vi "Main.vi"(11 "Module Admin":refnum<class "Delacor_lib_QMH_Module Admin.lvclass">) -> ()   [LabVIEW 2023, in "Panther Dashboard.lvlib"]
doc: "Panther Dashboard For DQMH®\n\nDeveloped and maintained by:\nPantherLAB\n\nMain Contributor- Developer:\n\n» Enrique Noé Arias\n\nBrainstorming & Code Reviews:\n\n» Matthias Baudot\n» Fabiola De La Cueva\n» Christopher Farmer\n» Cyril Gambini\n» Joerg Hampel\n» Olivier Jourdan\n» Cesar Muñoz\n» Darren Nattinger\n» Luis Orozco\n» Sam Taggart\n» Diego Torres"
uses:
  Panther Dashboard.lvlib
  <vilib>/Delacor/Delacor QMH/Libraries/Module Admin_class/Delacor_lib_QMH_Module Admin.lvclass
  Module Data--cluster.ctl
  Maps List and refs--cluster.ctl
  <vilib>/National Instruments/Tree Map/Tree Map Data.ctl
  DQMH Modules Info--cluster.ctl
  Module type--enum.ctl
  Project References--cluster.ctl
  Selection Type--enum.ctl
  References Updated Argument--cluster.ctl
  Launch DQMH Scripting Tools Argument--cluster.ctl
  DQMH Tools Menu--enum.ctl
  <vilib>/Delacor/Delacor QMH/Libraries/Message Queue_class/Delacor_lib_QMH_Message Queue.lvclass/Delacor_lib_QMH_Message Queue.ctl
  Expand Results Argument--cluster.ctl
  Execute Default Event Request Argument--cluster.ctl
  Tree DQMH Selection Argument--cluster.ctl
  Scan DQMH Modules Argument--cluster.ctl
  Stop Argument--cluster.ctl
  Generate Project Documentation Argument--cluster.ctl
  Set App Theme Argument--cluster.ctl
  Show About Argument--cluster.ctl
  Update Module ID Argument--cluster.ctl
  Save Library Description Argument--cluster.ctl
  Save VI Description Argument--cluster.ctl
  Open Documentation Argument--cluster.ctl
  Save Project Documentation Argument--cluster.ctl
  Public VIs names--enum.ctl
  <vilib>/Delacor/Delacor QMH/Libraries/Module Admin_class/Delacor_lib_QMH_Module Admin.lvclass/Delacor_lib_QMH_Module Admin.ctl
  <vilib>/Delacor/Delacor QMH/Libraries/Message Queue_class/Delacor_lib_QMH_Enqueue Message (Single).vi
  <vilib>/Delacor/Delacor QMH/Libraries/Module Admin_class/Delacor_lib_QMH_Get External Launch.vi
  Panther Dashboard--global.vi
  <vilib>/National Instruments/Tree Map/API/List Roots.vi
  <vilib>/National Instruments/Tree Map/Utility/Into Tree Control Items.vi
  <vilib>/Utility/error.llb/Error Cluster From Error Code.vi
  <vilib>/ErrorRing/Error Ring.xnode
  <vilib>/Delacor/Delacor QMH/Libraries/Message Queue_class/Delacor_lib_QMH_Message Queue.lvclass
  <vilib>/National Instruments/Tree Map/Tree Map.lvlib
  <vilib>/Delacor/Delacor QMH/Libraries/Scripting API/DQMH_Scripting API.lvlib
  ContextHelp/ContextHelp.lvlib
panel:
  out "error out":errorcluster
  in  "Context Help Panther":bool caption="Doc Editor"
  in  "Add Event":bool
  in  "Remove Event":bool caption="Remove"
  in  "Convert Event":bool caption="Convert"
  in  "Rename Event":bool caption="Rename"
  in  "Add New Module":bool caption="Add"
  in  "Rename Module":bool caption="Rename"
  in  "Validate Module":bool caption="Validate"
  in  "Create Module Template":bool caption="Template"
  in  "Add Unit Test Module":bool caption="Unit Test"
  in  "Create RT Tester Module":bool caption="RT Tester"
  in  "About Panther":bool caption="About"
  in  "Theme Panther":bool caption="Theme"
  in  "Projects":string(combo)
  in  "Targets":string(combo)
  in  "Search":bool caption="Scan Project"
  in  "Expand Results":bool
  in  "Include Dependencies":bool
  in  "Module ID":i32=-1 min=-1 max=1000 step=1 format="Module ID %d"
  in  "Modules Tree":string(tree) caption="Tree 2"
  out "Panther Indicator":bool
  out "Process Indicator":bool
  out "Event Indicator":bool
  out "Status":string
  out "Progress":u16(slide) scale=-1.0..4.0
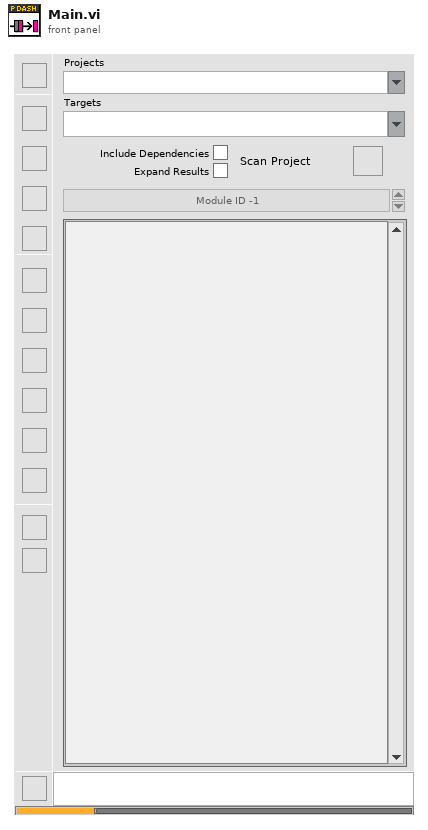
[diagram p1: front panel]
types:
  T1 = typedef "Panther Dashboard.lvlib/Broadcast Events--cluster.ctl" = cluster{"Module Did Init":refnum<user-event>, "Status Updated":refnum<user-event>, "Error Reported":refnum<user-event>, "Module Did Stop":refnum<user-event>, "Update Module Execution Status":refnum<user-event>, "References Updated":refnum<user-event>, "Projects Updated":refnum<user-event>, "Targets Updated":refnum<user-event>, "Progress updated":refnum<user-event>, "Scale Updated":refnum<user-event>, "Connector Pane Updated":refnum<user-event>, "Documentation Updated":refnum<user-event>, "Module Type Updated":refnum<user-event>, "Theme Updated":refnum<user-event>, "Project Description Updated":refnum<user-event>}
  T2 = typedef "Panther Dashboard.lvlib/Request Events--cluster.ctl" = cluster{"Stop Module":refnum<user-event>, "Show Panel":refnum<user-event>, "Hide Panel":refnum<user-event>, "Get Module Execution Status":refnum<user-event>, "Show Diagram":refnum<user-event>, "Scan DQMH Modules":refnum<user-event>, "Tree DQMH Selection":refnum<user-event>, "Open Module API Tester":refnum<user-event>, "Execute Default Event Request":refnum<user-event>, "Expand Results":refnum<user-event>, "Launch DQMH Scripting Tools":refnum<user-event>, "Generate Project Documentation":refnum<user-event>, "Set App Theme":refnum<user-event>, "Show About":refnum<user-event>, "Update Module ID":refnum<user-event>, "Save Library Description":refnum<user-event>, "Save VI Description":refnum<user-event>, "Open Documentation":refnum<user-event>, "Save Project Documentation":refnum<user-event>, "Register controls Mouse Enter":refnum<user-event>}
  T3 = typedef "ContextHelp.lvlib/Broadcast Events--cluster.ctl" = cluster{"Module Did Init":refnum<user-event>, "Status Updated":refnum<user-event>, "Error Reported":refnum<user-event>, "Module Did Stop":refnum<user-event>, "Update Module Execution Status":refnum<user-event>}
  T4 = typedef "Panther Dashboard.lvlib/Selection Type--enum.ctl" = enum16{"Broadcast", "Request", "Module", "Public API"}
  T5 = typedef "Panther Dashboard.lvlib/Module Data--cluster.ctl" = cluster{"Maps":T6, "DQMH Scan Results":T8, "Current Selection":cluster{"VI Ref":refnum<vi>, "DQMH Lib Ref":refnum<vi>}, "Module type":T9, "Module ID":i32, "Theme":bool, "Broadcast?":bool}
  T6 = typedef "Panther Dashboard.lvlib/Maps List and refs--cluster.ctl" = cluster{"Tree Map":T7, "References Map":map{string, refnum<vi>}}
  T7 = typedef "Tree Map.lvlib/Tree Map Data.ctl" = map{string, cluster{"Child Paths Set":set{string}, "Name":string, "Data":string, "Attributes":map{string, string}}}
  T8 = typedef "Panther Dashboard.lvlib/DQMH Modules Info--cluster.ctl" = cluster{"All DQMH Modules Refs":refnum<vi>[], "All Modules Descriptions":string[], "All Modules type":T9[], "Project References":T10}
  T9 = typedef "Panther Dashboard.lvlib/Module type--enum.ctl" = enum16{"Module type: Singleton", "Module type: Cloneable"}
  T10 = typedef "Panther Dashboard.lvlib/Project References--cluster.ctl" = cluster{"Project Ref":refnum<vi>, "Project Name":string, "Target":refnum<vi>, "App Ref":refnum<vi>}
  T11 = typedef "Panther Dashboard.lvlib/References Updated Argument--cluster.ctl" = cluster{"Modules":refnum<vi>[], "Modules Types":T9[], "Application Instance":refnum<vi>}
  T12 = enum8{"Enabled", "Disabled", "Disabled and Grayed Out"}
  T13 = typedef "Panther Dashboard.lvlib/Launch DQMH Scripting Tools Argument--cluster.ctl" = cluster{"Scripting Tool":T14}
  T14 = typedef "Panther Dashboard.lvlib/DQMH Tools Menu--enum.ctl" = enum16{"Create New DQMH Event", "Remove DQMH Event", "Convert DQMH Event", "Rename DQMH Event", "Add New DQMH Module", "Create RT Tester", "Rename DQMH Module", "Validate DQMH Module", "Create DQMH Module Template", "New DQMH  Unit Test"}
  T15 = typedef "Panther Dashboard.lvlib/Expand Results Argument--cluster.ctl" = cluster{"Expand?":bool}
  T16 = typedef "Panther Dashboard.lvlib/Execute Default Event Request Argument--cluster.ctl" = cluster{"Event Name":string}
  T17 = typedef "Panther Dashboard.lvlib/Tree DQMH Selection Argument--cluster.ctl" = cluster{"Tree DQMH Sel":string}
  T18 = typedef "Panther Dashboard.lvlib/Scan DQMH Modules Argument--cluster.ctl" = cluster{"Include Dependencies":bool, "Project":string, "Target":string}
  T19 = enum32{"invalid lock state", "Not Locked", "Locked (No Password)", "Password-protected"}
  T20 = typedef "Panther Dashboard.lvlib/Stop Argument--cluster.ctl" = cluster{"Origin":string, "Exit via Stop Module Req?":bool, "Wait for Module to stop?":bool}
  T21 = typedef "Panther Dashboard.lvlib/Generate Project Documentation Argument--cluster.ctl" = cluster{"Boolean":bool}
  T22 = typedef "Panther Dashboard.lvlib/Set App Theme Argument--cluster.ctl" = cluster{"Theme":bool}
  T23 = typedef "Panther Dashboard.lvlib/Show About Argument--cluster.ctl" = cluster{"Boolean":bool}
  T24 = typedef "Panther Dashboard.lvlib/Update Module ID Argument--cluster.ctl" = cluster{"New ID":i32}
  T25 = typedef "Panther Dashboard.lvlib/Save Library Description Argument--cluster.ctl" = cluster{"Library Description":string}
  T26 = typedef "Panther Dashboard.lvlib/Save VI Description Argument--cluster.ctl" = cluster{"VI Description":string}
  T27 = typedef "Panther Dashboard.lvlib/Open Documentation Argument--cluster.ctl" = cluster{"Boolean":bool}
  T28 = typedef "Panther Dashboard.lvlib/Save Project Documentation Argument--cluster.ctl" = cluster{"Project Description":string}
  T29 = typedef "Panther Dashboard.lvlib/Public VIs names--enum.ctl" = enum16{"Start Module.vi", "Synchronize Module Events.vi", "Obtain Broadcast Events for Registration.vi", "Null Broadcast Events--constant.vi", "Stop Module.vi"}
  T30 = cluster{"Left Cell String":string, "Child Text":string[], "Child Tag":string, "Item Indent":i32, "Child Only?":bool, "Glyph Index":i32}[]
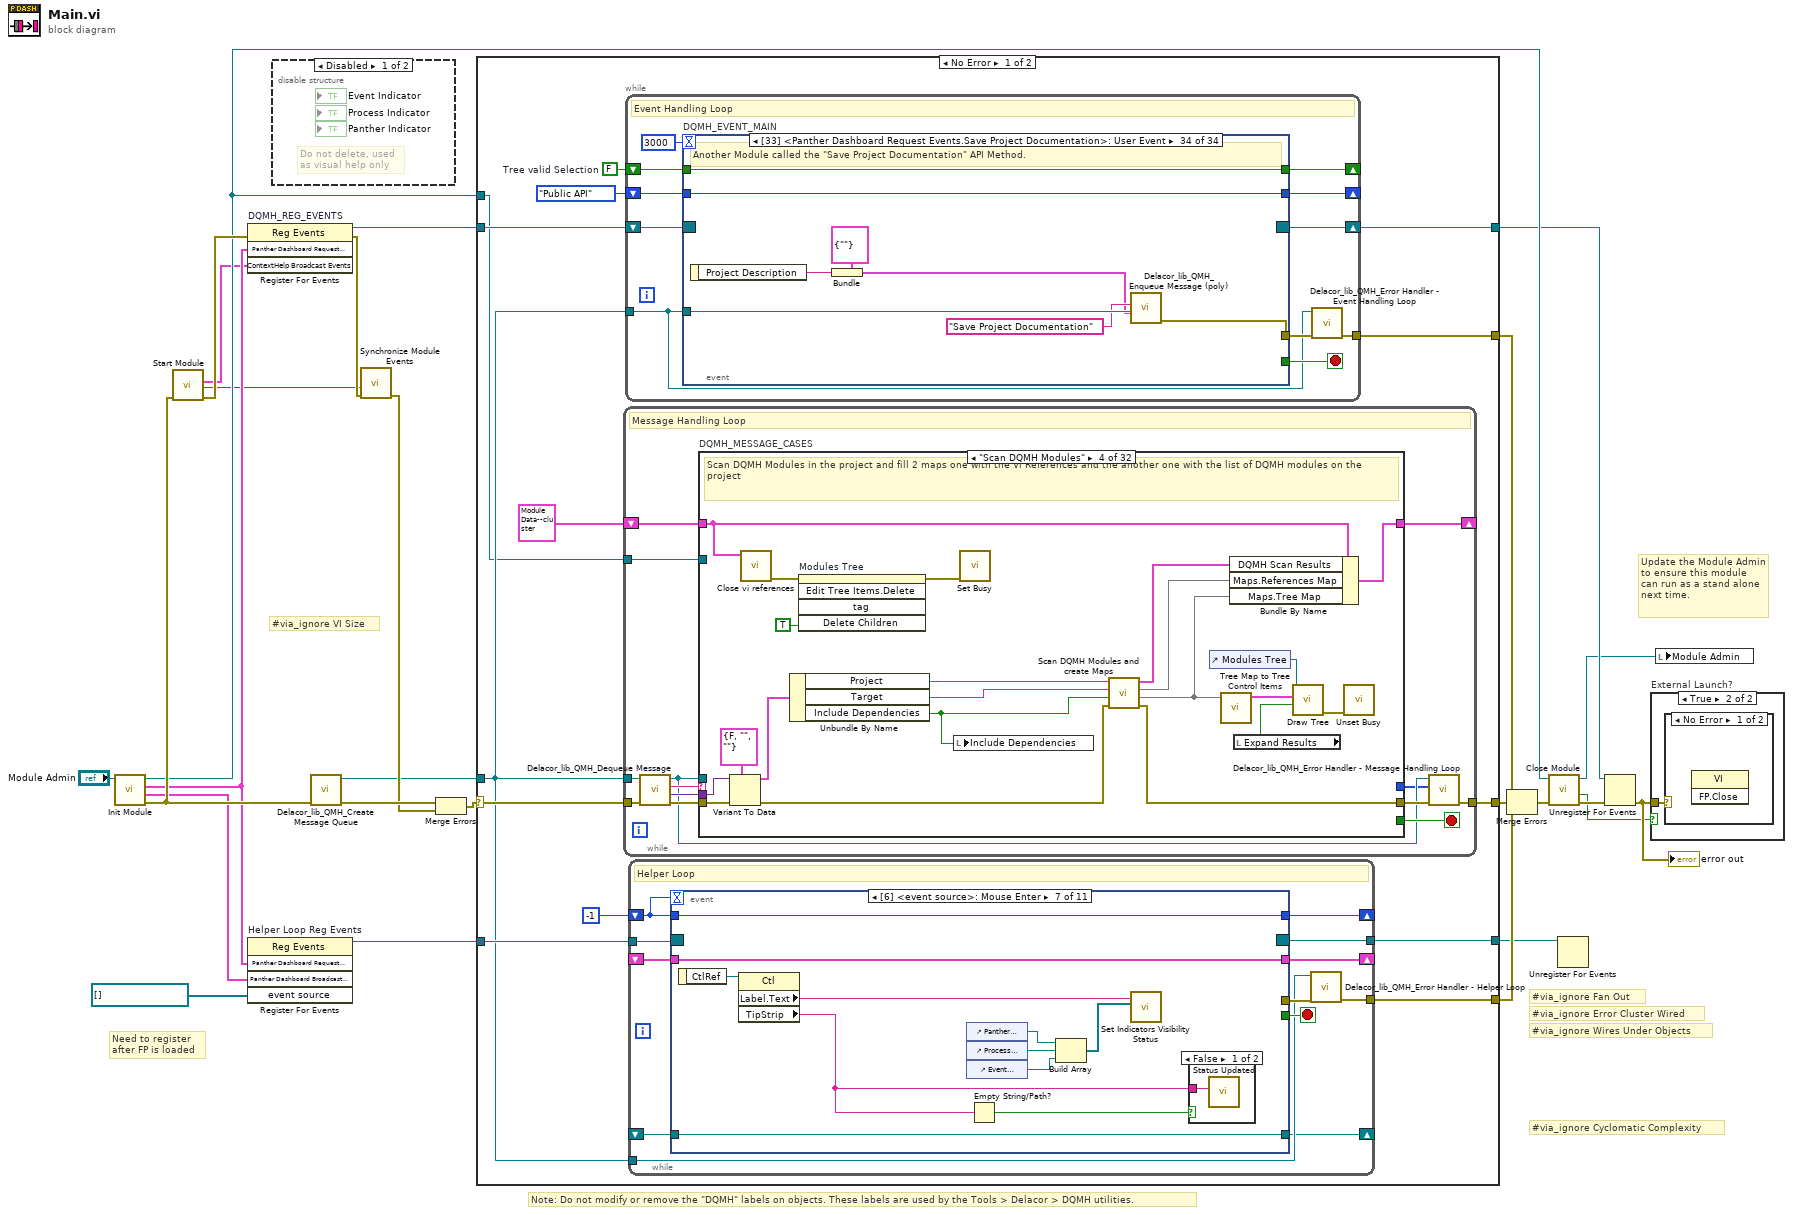
[diagram p0: block diagram]
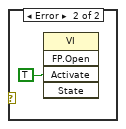
[diagram p4: hidden frame]
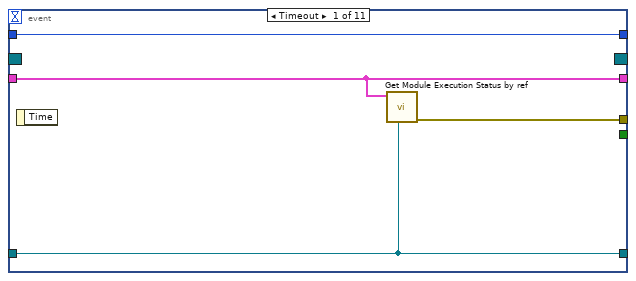
[diagram p5: hidden frame]
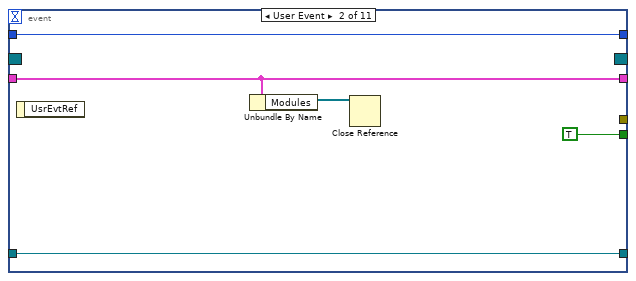
[diagram p6: hidden frame]
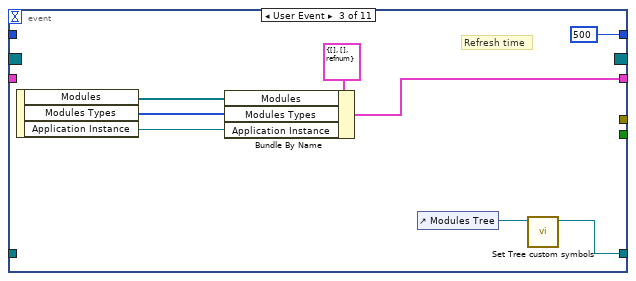
[diagram p7: hidden frame]
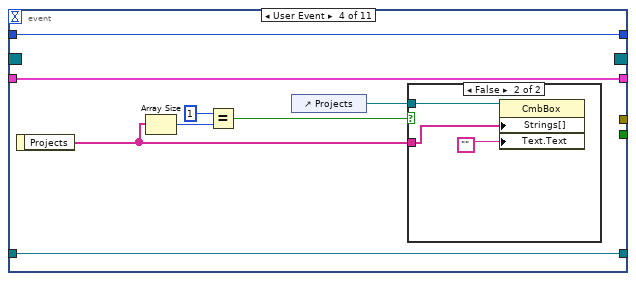
[diagram p8: hidden frame]
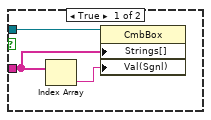
[diagram p9: hidden frame]
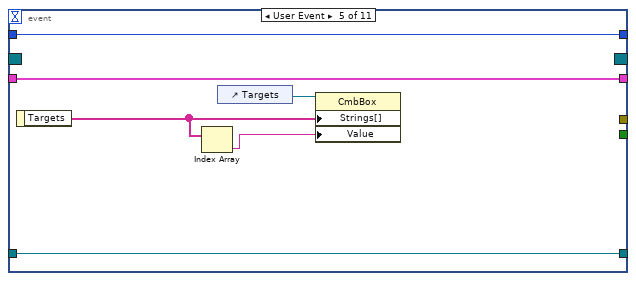
[diagram p10: hidden frame]
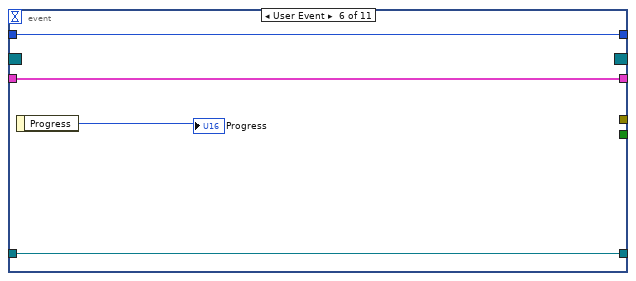
[diagram p11: hidden frame]
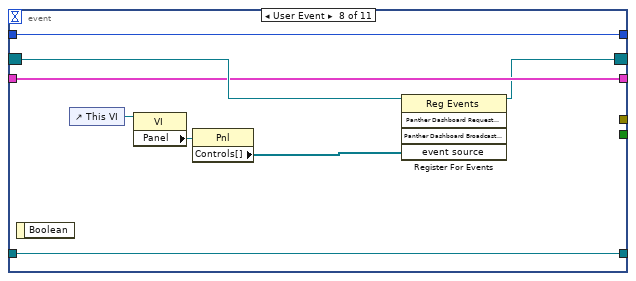
[diagram p13: hidden frame]
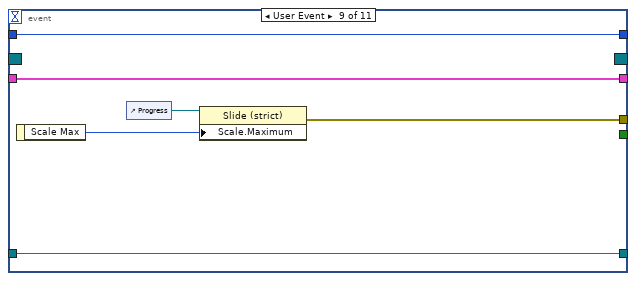
[diagram p14: hidden frame]
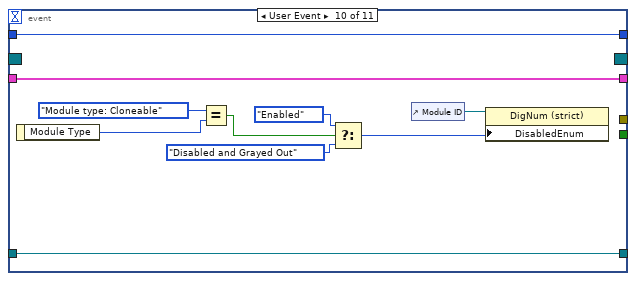
[diagram p15: hidden frame]
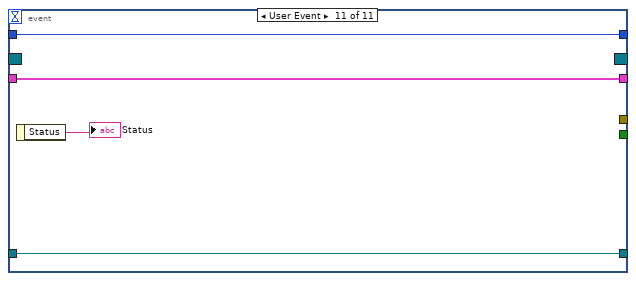
[diagram p16: hidden frame]
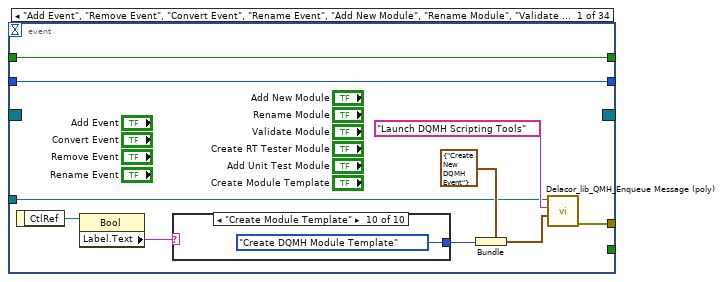
[diagram p17: hidden frame]
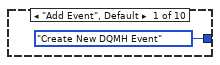
[diagram p18: hidden frame]
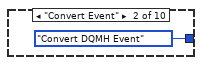
[diagram p19: hidden frame]
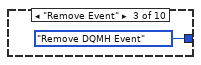
[diagram p20: hidden frame]
diagram:
  # "Need to register\nafter FP is loaded"
  # "#via_ignore VI Size"
  # "#via_ignore Fan Out"
  # "#via_ignore Cyclomatic Complexity"
  # "#via_ignore Wires Under Objects"
  # "#via_ignore Error Cluster Wired"
  # "Note: Do not modify or remove the \"DQMH\" labels on objects. These labels are used by the Tools > Delacor > DQMH utilities."
  # "Update the Module Admin to ensure this module can run as a stand alone next time."
  n1 = call "Init Module.vi"("Singleton Module Admin in"="Module Admin") -> ("error out"=w15:errorcluster, "Panther Dashboard Broadcast Events"=w4:T1, "Panther Dashboard Request Events"=w5:T2, "Singleton Module Admin out"=w14:refnum<class "Delacor_lib_QMH_Module Admin.lvclass">)  [unwired: 7 in]
  n2 = call "Start Module.vi"("error in"=w15) -> ("error out"=w17:errorcluster, "Wait for Event Sync?"=w3:bool, "ContextHelp Broadcast Events"=w2:T3)  [unwired: 7 in, 1 out]
  n3 = register-events "DQMH_REG_EVENTS"(error in=w17, w5, w2) -> (reference out=w12:refnum<event-registration>, error out=w18:errorcluster)  [unwired: 1 in]
  n4 = register-events "Helper Loop Reg Events"(w5, w4, refnum<vi>[] [] ("event source")) -> (reference out=w7:refnum<event-registration>)  [unwired: 2 in, 1 out]
  n5 = disable-structure shown="Disabled" {
    frame Disabled {
      # "Do not delete, used\nas visual help only"
    }
    frame Enabled {
    }
  }
  n6 = call <vilib>:"Delacor_lib_QMH_Create Message Queue.vi"("error in"=w15) -> ("error out"=w21:errorcluster, "Message Queue"=w11:refnum<class "Delacor_lib_QMH_Message Queue.lvclass">)  [unwired: 9 in]
  n7 = call "Synchronize Module Events.vi"("error in"=w18, "Wait for Event Sync?"=w3) -> ("error out"=w16:errorcluster)  [unwired: 9 in]
  n8 = Merge Errors(w21, w16) -> (w20:errorcluster)
  n9 = case shown="No Error" w20 {
    selector: w20 -> [w38 w777]
    tunnel: [w40 w776] -> w26
    tunnel: [w36 w775] -> w13
    tunnel: w12 -> [w34 w775]
    tunnel: w11 -> [w30 w771]
    tunnel: [w39 _] -> w24
    tunnel: w14 -> [w27 w772]
    tunnel: w7 -> [w33 w770]
    tunnel: [w32 w770] -> w6
    tunnel: [w37 _] -> w19
    frame No Error {
      w29 = FALSE  # Tree valid Selection
      n10 = while {
        tunnel: w30 -> [w428]
        shift-right: [w432] -> _
        shift-left: T5 {"Maps"={"Tree Map"={}, "References Map"={}}, "DQMH Scan Results"={"All DQMH Modules Refs"=[], "All Modules Descriptions"=[], "All Modules type"=[], "Project References"={"Project Ref"=refnum, "Project Name"="", "Target"=refnum, "App Ref"=refnum}}, "Current Selection"={"VI Ref"=refnum, "DQMH Lib Ref"=refnum}, "Module type"=enum."Module type: Singleton", "Module ID"=0, "Theme"=FALSE, "Broadcast?"=FALSE} ("Data Cluster") -> [w433]
        tunnel: w38 -> [w436]
        tunnel: [w434] -> w40
        tunnel: w27 -> [w426]
        stop <- w431 stop-if-true
        # "Message Handling Loop"
        n11 = call-dynamic "Delacor_lib_QMH_Dequeue Message.vi"("error in"=w436, "Message Queue in"=w428) -> ("error out"=w435:errorcluster, "Message Data"=w429:variant, "Message"=w430:string, "Message Queue out"=w427:refnum<class "Delacor_lib_QMH_Message Queue.lvclass">)  [unwired: 6 in]
        n12 = case "DQMH_MESSAGE_CASES" shown="\"Scan DQMH Modules\"" w430 {
          selector: w430 -> [_ w465 _ _ _ _ _ _ _ _ _ _ _ _ _ _ _ _ _ _ _ _ _ _ _ _ _ _ _ _ _ w756]
          tunnel: w427 -> [_ _ _ _ _ _ _ _ _ _ _ _ _ _ _ _ _ _ _ _ _ _ _ _ _ _ _ _ _ w725 w748 _]
          tunnel: w435 -> [w459 w470 w472 w493 w500 w507 w514 w521 w536 w545 w550 w556 w570 w583 w605 w611 w613 w625 w632 w637 w650 w661 w670 w678 w688 w704 w717 w720 w722 w732 w754 w758]
          tunnel: [w453 w468 w472 w492 w499 w507 w514 w521 w535 w544 w551 w557 w568 w581 w606 w610 w614 w624 w631 w636 w648 w658 w666 w677 w686 w702 w715 w719 w722 w728 w751 w759] -> w437
          tunnel: w433 -> [w438 w467 w471 w479 w497 w506 w513 w520 w531 w543 w549 w555 w563 w580 w604 w609 w618 w623 w630 w635 w639 w657 w665 w676 w680 w697 w711 w718 w721 w727 w740 w757]
          tunnel: [w450 w467 w471 w484 w497 w506 w513 w520 w527 w543 w549 w555 w563 w580 w604 w609 w618 w621 w630 w635 w639 w652 w665 w672 w679 w695 w711 w718 w721 w727 w740 w757] -> w432
          tunnel: [_ _ _ _ _ _ _ _ _ _ _ _ _ _ _ _ _ _ _ _ _ _ _ _ _ _ _ _ _ _ w747 _] -> w431
          tunnel: w429 -> [_ w466 _ w487 _ _ _ _ w534 _ _ _ w566 _ _ _ _ w622 w629 _ w647 w656 w664 w675 w684 w700 w714 _ _ w726 w746 _]
          tunnel: w426 -> [w451 _ _ _ _ _ _ _ _ _ _ _ _ _ _ _ _ _ _ _ _ _ _ _ _ _ _ _ _ w724 w741 _]
          tunnel: [_ _ _ _ _ _ _ _ _ _ _ _ _ i32[] [5000, 1026, 43] ("specific error code to clear (0: all)") _ _ _ _ _ _ _ _ _ _ _ _ _ _ _ _ _ _] -> w425
          frame "Initialize" {
            w441 = "Panther Dashboard for DQMH" ("format string")
            # "Initialize - Any operation that needs to be done before the module can receive messages. Synchronize Caller Events.vi will inform Start Module.vi that the module has launched and is ready to receive messages. Module Did Init.vi will broadcast that the module initialized."
            n13 = call "Synchronize Caller Events.vi"("error in (no error)"=w459, "Singleton Module Admin in"=w451) -> ("error out"=w458:errorcluster)  [unwired: 8 in, 1 out]
            n14 = call "Module Name--constant.vi"() -> ("Module Name"=w448:string)  [unwired: 11 in]
            n15 = disable-structure shown="Disabled" {
              disable-tunnel: [w462 _] -> w439
              disable-tunnel: w438 -> [w461 _]
              frame Disabled {
                n16 = call "Close vi references.vi"("Data Cluster"=w461) -> ("error out"=w460:errorcluster)  [unwired: 10 in]
                n17 = invoke on="Modules Tree" class="Tree (strict)" method="Edit Tree Items.Delete"(error in=w460) -> (error out=w462:errorcluster)  [unwired: 4 in, 4 out]
              }
              frame Enabled {
              }
            }
            n18 = call "Module Did Init.vi"("error in (no error)"=w458, "Initialized?"=TRUE, "Origin"=w448) -> ("error out"=w457:errorcluster)  [unwired: 8 in]
            n19 = property on="Modules Tree" class="Tree (strict)"(error in=w439, "Allow Item Drag"=TRUE ("Drag/Drop:Allow Dragging"), "SelColor"=u32 8355711) -> ()  [unwired: 1 in, 2 out]
            n20 = control-ref of="Projects"() -> (w444:refnum<vi>)
            n21 = call "Scan For App Projects.vi"("error in"=w457, "Init?"=TRUE, "Projects Ref"=w444) -> ("error out"=w456:errorcluster)  [unwired: 8 in]
            n22 = call "Read Theme from Config.vi"("error in"=w456) -> ("error out"=w455:errorcluster, "Theme"=w440:bool)  [unwired: 9 in]
            n23 = local write "Theme Panther"(w440) -> ()
            n24 = call "Set App Theme.vi"("error in"=w455, "Theme"=w440) -> ("error out"=w454:errorcluster)  [unwired: 9 in]
            n25 = control-ref of="This VI"() -> (w442:refnum<vi>)
            n26 = Bundle By Name(cluster=w438, "Module ID"=-1) -> (w450:T5)
            n27 = call "Status Updated.vi"("Status"=w441) -> ()  [unwired: 10 in, 1 out]
            n28 = call "Set Panel Initial State.vi"("Title"=w441, "Main Vi Ref"=w442) -> ("error out"=w452:errorcluster)  [unwired: 9 in]
            n29 = Merge Errors(w452, w454) -> (w453:errorcluster)
          }
          frame "Refresh Targets" {
            # "When the User selects a Project triggers this task to scan all the targets available"
            n30 = Variant To Data(error in=w470, type=w465, Variant=w466) -> (data=w464:string, error out=w469:errorcluster)
            n31 = call "Get all Targets.vi"("error in"=w469, "Project Selection"=w464) -> ("error out"=w468:errorcluster, "Targets"=w463:string[])  [unwired: 8 in]
            n32 = call "Targets Updated.vi"("Targets"=w463) -> ()  [unwired: 10 in, 1 out]
          }
          frame "---Module Specific---" {
            # "Separator -- The following cases handle messages specific to this Module."
          }
          frame "Scan DQMH Modules" {
            # "Scan DQMH Modules in the project and fill 2 maps one with the Vi References and the another one with the list of DQMH modules on the project"
            n33 = Variant To Data(error in=w493, type=T18 {"Include Dependencies"=FALSE, "Project"="", "Target"=""} ("Scan DQMH Modules Argument"), Variant=w487) -> (data=w485:T18, error out=w490:errorcluster)
            n34 = call "Close vi references.vi"("Data Cluster"=w479) -> ("error out"=w489:errorcluster)  [unwired: 10 in]
            n35 = Unbundle By Name(w485) -> ("Project"=w475:string, "Target"=w477:string, "Include Dependencies"=w478:bool)
            n36 = invoke on="Modules Tree" class="Tree (strict)" method="Edit Tree Items.Delete"(error in=w489, "Delete Children"=TRUE ("Delete Children?")) -> (error out=w488:errorcluster)  [unwired: 3 in, 4 out]
            n37 = local write "Include Dependencies"(w478) -> ()
            n38 = call <vilib>:"Set Busy.vi"("error in (no error)"=w488) -> ()  [unwired: 9 in, 2 out]
            n39 = call "Scan DQMH Modules and create Maps.vi"("error in"=w490, "Include Dependencies"=w478, "Target Selection"=w477, "Project"=w475) -> ("error out"=w492:errorcluster, "Tree Map out"=w476:T7, "map ref out"=w480:map{string, refnum<vi>}, "DQMH Scan Results"=w483:T8)  [unwired: 4 in]
            n40 = control-ref of="Modules Tree"() -> (w481:refnum<vi>)
            n41 = call <vilib>:"Tree Map to Tree Control Items.vi"("Tree Map In"=w476) -> ("Tree Control Items"=w482:T30)  [unwired: 10 in]
            n42 = Bundle By Name(cluster=w479, "DQMH Scan Results"=w483, "Maps.References Map"=w480, "Maps.Tree Map"=w476) -> (w484:T5)
            n43 = local read "Expand Results"() -> (w473:bool)
            n44 = call "Draw Tree.vi"("Expanded Results?"=w473, "Tree Control Items"=w482, "TreeControl in"=w481) -> ("error out"=w491:errorcluster)  [unwired: 8 in]
            n45 = call <vilib>:"Unset Busy.vi"("error in (no error)"=w491) -> ()  [unwired: 10 in, 1 out]
          }
          frame "Drag VI" {
            # "This is the functionality alowing drag and drop the current selection to your code, you can build code using panther Dashboard."
            n46 = Unbundle By Name(w497) -> ("DQMH Scan Results.Project References.App Ref"=w496:refnum<vi>, "DQMH Scan Results.Project References.Target"=w495:refnum<vi>, "Current Selection.VI Ref"=w494:refnum<vi>)
            n47 = call "Drop Event into subVI.vi"("Current Selection.VI Ref"=w494, "Target"=w495, "App Ref"=w496) -> ("error out"=w498:errorcluster)  [unwired: 8 in]
            n48 = Merge Errors(w498, w500) -> (w499:errorcluster)
          }
          frame "Who is launching this module?" {
            # "Find all the VIS calling the Start Module.vi of the selected module library"
            n49 = Unbundle By Name(w506) -> ("Theme"=w505:bool, "DQMH Scan Results.Project References.App Ref"=w504:refnum<vi>, "DQMH Scan Results.Project References.Target"=w503:refnum<vi>, "Current Selection.DQMH Lib Ref"=w502:refnum<vi>)
            n50 = call "Find some Public API VI.vi"("Theme"=w505, "Framework VI to Find"=Public_VIs_names--enum."Start Module.vi", "Library in"=w502, "Target"=w503, "App Ref"=w504) -> ()  [unwired: 7 in]
          }
          frame "Who is registered to this module's broadcasts?" {
            # "Find all the VIS calling the Obtain broadcast events for registration of the selected module library"
            n51 = Unbundle By Name(w513) -> ("Theme"=w511:bool, "DQMH Scan Results.Project References.App Ref"=w510:refnum<vi>, "DQMH Scan Results.Project References.Target"=w509:refnum<vi>, "Current Selection.DQMH Lib Ref"=w508:refnum<vi>)
            n52 = call "Find some Public API VI.vi"("Theme"=w511, "Framework VI to Find"=Public_VIs_names--enum."Obtain Broadcast Events for Registration.vi", "Library in"=w508, "Target"=w509, "App Ref"=w510) -> ()  [unwired: 7 in]
          }
          frame "Who is stopping this module?" {
            # "Find all the VIS calling the Obtain broadcast events for registration of the selected module library"
            n53 = Unbundle By Name(w520) -> ("Theme"=w518:bool, "DQMH Scan Results.Project References.App Ref"=w517:refnum<vi>, "DQMH Scan Results.Project References.Target"=w516:refnum<vi>, "Current Selection.DQMH Lib Ref"=w515:refnum<vi>)
            n54 = call "Find some Public API VI.vi"("Theme"=w518, "Framework VI to Find"=Public_VIs_names--enum."Stop Module.vi", "Library in"=w515, "Target"=w516, "App Ref"=w517) -> ()  [unwired: 7 in]
          }
          frame "Tree DQMH Selection" {
            # "There is a new selection of the DQMH Tree list, need to search and update indicators acordanly."
            n55 = Unbundle By Name(w531) -> ("Maps.Tree Map"=w530:T7, "Maps.References Map"=w529:map{string, refnum<vi>}, "DQMH Scan Results"=w528:T8)
            n56 = Variant To Data(error in=w536, type=T17 {"Tree DQMH Sel"=""} ("Tree DQMH Selection Argument"), Variant=w534) -> (data=w532:T17, error out=w535:errorcluster)
            n57 = Unbundle By Name(w532) -> ("Tree DQMH Sel"=w524:string)
            n58 = call "Get List Information.vi"("List Selection"=w524, "DQMH Scan Info"=w528, "References Map"=w529, "Tree Map"=w530) -> ("Broadcast?"=w522:bool, "Vi out"=w525:refnum<vi>, "Module type"=w523:T9, "DQMH Lib"=w526:refnum<vi>)  [unwired: 4 in]
            n59 = Bundle By Name(cluster=w531, "Current Selection.DQMH Lib Ref"=w526, "Current Selection.VI Ref"=w525, "Module type"=w523, "Broadcast?"=w522) -> (w527:T5)
          }
          frame "Open Module API Tester" {
            # "If nothing selected use the first DQMH module"
            # "Open the API Tester from the current DQMH Module Selected"
            n60 = Unbundle By Name(w543) -> ("DQMH Scan Results.Project References.App Ref"=w542:refnum<vi>, "DQMH Scan Results.All DQMH Modules Refs"=w541:refnum<vi>[], "Current Selection.DQMH Lib Ref"=w537:refnum<vi>)
            n61 = Index Array(array=w541) -> (element=w539:refnum<vi>)  [unwired: 1 in]
            n62 = Not A Number/Path/Refnum?(number/path/refnum=w537) -> (NaN/Path/Refnum?=w540:bool)
            n63 = Select(t=w539, s=w540, f=w537) -> (s? t:f=w538:refnum<vi>)
            n64 = call "Open API Tester.vi"("error in"=w545, "DQMH Library Ref"=w538, "Application Instance"=w542) -> ("error out"=w544:errorcluster)  [unwired: 8 in]
          }
          frame "Find Module in project" {
            # "Find the selected module in project explorer"
            n65 = Unbundle By Name(w549) -> ("Current Selection.DQMH Lib Ref"=w548:refnum<vi>, "DQMH Scan Results.Project References.Project Ref"=w547:refnum<vi>, "DQMH Scan Results.All DQMH Modules Refs"=w546:refnum<vi>[])
            n66 = call "Find Library in Project.vi"("error in (no error)"=w550, "DQMH Modules Refs"=w546, "Project Ref"=w547, "DQMH Lib Ref"=w548) -> ("error out"=w551:errorcluster)  [unwired: 7 in]
          }
          frame "Locate Event on Main" {
            # "Find the selected event vi on the owing DQMH Module, if it is a reques we highlight its frame, if it is a broadcast we highlight where the broadcast is being triggered"
            n67 = Unbundle By Name(w555) -> ("DQMH Scan Results.Project References.App Ref"=w553:refnum<vi>, "Current Selection.VI Ref"=w554:refnum<vi>, "Broadcast?"=w552:bool)
            n68 = call "Find Event Frame.vi"("error in"=w556, "Broadcast?"=w552, "VI in"=w554, "Application Instance"=w553) -> ("error out"=w557:errorcluster)  [unwired: 7 in]
          }
          frame "Execute Default Event Request" {
            # "Execute Default Event"
            n69 = Variant To Data(error in=w570, type=T16 {"Event Name"=""} ("Execute Default Event Request Argument"), Variant=w566) -> (data=w564:T16, error out=w569:errorcluster)
            n70 = Unbundle By Name(w563) -> ("DQMH Scan Results.Project References.App Ref"=w562:refnum<vi>, "Current Selection.DQMH Lib Ref"=w561:refnum<vi>, "Module ID"=w559:i32, "Module type"=w558:T9)
            n71 = Unbundle By Name(w564) -> ("Event Name"=w560:string)
            n72 = call "Execute Default event.vi"("Module type"=w558, "Module ID"=w559, "Event"=w560, "DQMH Library Ref"=w561, "application Instance"=w562) -> ("error out"=w567:errorcluster)  [unwired: 6 in]
            n73 = Merge Errors(w569, w567) -> (w568:errorcluster)
          }
          frame "Search for Event Callers / listeners" {
            # "1026-Invalid Ref\n43- Operation\n canceled by user\n5000- something\nrandom happening\non DQMH Scripting\nAPI"
            # "Search for this event callers"
            n74 = Unbundle By Name(w580) -> ("DQMH Scan Results.Project References.Project Ref"=w574:refnum<vi>, "Current Selection.VI Ref"=w579:refnum<vi>, "Theme"=w571:bool, "Broadcast?"=w572:bool)
            n75 = Select(t="Searching code registered to broadcast selection" ("Status"), s=w572, f="Searching for Event Callers" ("Status")) -> (s? t:f=w575:string)
            n76 = call "Status Updated.vi"("error in (no error)"=w583, "Status"=w575) -> ("error out"=w582:errorcluster)  [unwired: 9 in]
            n77 = case shown="False" w572 {
              tunnel: w582 -> [w588 w595]
              tunnel: [w587 w594] -> w581
              tunnel: w579 -> [w586 w591]
              tunnel: [w585 w593] -> w578
              tunnel: w574 -> [w584 w592]
              frame False {
                # "Requests"
                n78 = call <vilib>:"Get Callers of Request VI in Project.vi"("error in"=w588, "Request VI"=w586, "Project"=w584) -> ("error out"=w587:errorcluster, "Request VI Callers"=w585:refnum<vi>[])  [unwired: 7 in]
              }
              frame True {
                # "Broadcast"
                n79 = Two Button Dialog(message="This is an exhaustive task that can take up to minutes, do you wish to continue?") -> (T button?=w590:bool)  [unwired: 2 in]
                n80 = case shown="False" w590 {
                  tunnel: w595 -> [w596 w601]
                  tunnel: [w596 w600] -> w594
                  tunnel: [_ w599] -> w593
                  tunnel: w592 -> [_ w598]
                  tunnel: w591 -> [_ w597]
                  frame False {
                  }
                  frame True {
                    n81 = call <vilib>:"Get VIs Registered for Broadcast in Project.vi"("error in"=w601, "Broadcast VI"=w597, "Project"=w598) -> ("error out"=w600:errorcluster, "VIs Registered for Broadcast"=w599:refnum<vi>[])  [unwired: 7 in]
                  }
                }
              }
            }
            n82 = call <vilib>:"Set Busy.vi"("error in (no error)"=w582) -> ()  [unwired: 9 in, 2 out]
            n83 = call <vilib>:"Unset Busy.vi"("error in (no error)"=w581) -> ()  [unwired: 10 in, 1 out]
            n84 = call "Start Call to results window.vi"("Find Broadcast?"=w572, "Request VI Callers"=w578, "Event"=w579, "Theme"=w571) -> ()  [unwired: 8 in]
          }
          frame "Open VI on Disk" {
            # "Open current event selection on the file system"
            n85 = Unbundle By Name(w604) -> ("Current Selection.VI Ref"=w603:refnum<vi>)
            n86 = property class="VI"(reference=w603) -> ("Path"=w602:path)  [unwired: 1 in, 2 out]
            n87 = call "Open File on Disk.vi"("error in"=w605, "file or directory path"=w602) -> ("error out"=w606:errorcluster)  [unwired: 9 in]
          }
          frame "Open File Library on Disk" {
            # "Open current Module Library selection on the file system"
            n88 = Unbundle By Name(w609) -> ("Current Selection.DQMH Lib Ref"=w608:refnum<vi>)
            n89 = property class="Library"(reference=w608) -> ("Path"=w607:path)  [unwired: 1 in, 2 out]
            n90 = call "Open File on Disk.vi"("error in"=w611, "file or directory path"=w607) -> ("error out"=w610:errorcluster)  [unwired: 9 in]
          }
          frame "Open Event Arguments" {
            # "Open The event selected DQMH Arguments, also open the Event BD to do edits on it"
            n91 = Unbundle By Name(w618) -> ("Current Selection.VI Ref"=w617:refnum<vi>)
            n92 = property on="Property Node" class="VI"(reference=w617, error in=w613, "BDWin.Open"=TRUE ("Block Diagram Window:Open")) -> (reference out=w615:refnum<vi>, error out=w612:errorcluster)
            n93 = call "Open Event Arguments.vi"("error in (no error)"=w612, "VI Refnum"=w615) -> ("error out"=w614:errorcluster)  [unwired: 9 in]
          }
          frame "Module ID Update" {
            # "Module ID Control has value change"
            n94 = Variant To Data(error in=w625, type=0 ("Module ID"), Variant=w622) -> (data=w620:i32, error out=w624:errorcluster)
            n95 = Bundle By Name(cluster=w623, "Module ID"=w620) -> (w621:T5)
          }
          frame "Expand or Close" {
            # "Expand or Close DQMH Tree control"
            n96 = Variant To Data(error in=w632, type=T15 {"Expand?"=FALSE} ("Expand or Close Argument"), Variant=w629) -> (data=w627:T15, error out=w631:errorcluster)
            n97 = Unbundle By Name(w627) -> ("Expand?"=w626:bool)
            n98 = invoke on="Modules Tree" class="Tree (strict)" method="Open/Close.Open/Close All"("Open"=w626) -> ()  [unwired: 3 in, 4 out]
          }
          frame "Open Project Folder" {
            n99 = Unbundle By Name(w635) -> ("DQMH Scan Results.Project References.Project Ref"=w634:refnum<vi>)
            n100 = property class="Project"(reference=w634) -> ("Path"=w633:path)  [unwired: 1 in, 2 out]
            n101 = call "Open File on Disk.vi"("error in"=w637, "file or directory path"=w633) -> ("error out"=w636:errorcluster)  [unwired: 9 in]
          }
          frame "Launch DQMH Scripting Tools" {
            # "Launch the DQMH Scripting Tools"
            n102 = Variant To Data(error in=w650, type=T13 {"Scripting Tool"=enum."Create New DQMH Event"} ("Launch DQMH Scripting Tools Argument"), Variant=w647) -> (data=w645:T13, error out=w649:errorcluster)
            n103 = Unbundle By Name(w645) -> ("Scripting Tool"=w640:T14)
            n104 = Unbundle By Name(w639) -> ("DQMH Scan Results.Project References.Project Name"=w643:string, "DQMH Scan Results.Project References.App Ref"=w644:refnum<vi>, "Current Selection.DQMH Lib Ref"=w638:refnum<vi>)
            n105 = Format Into String(format string="DQMH Tool: %s being executed ", w640) -> (resulting string=w642:string)  [unwired: 2 in, 1 out]
            n106 = call "Status Updated.vi"("Status"=w642) -> ()  [unwired: 10 in, 1 out]
            n107 = call "Launch DQMH Tools by menu.vi"("Project"=w643, "Application Instance"=w644, "error in"=w649, "Module Ref"=w638, "DQMH Tools"=w640) -> ("error out"=w648:errorcluster)  [unwired: 6 in]
          }
          frame "Set App Theme" {
            # "Set Panther Dashboard Theme"
            n108 = Variant To Data(error in=w661, type=T22 {"Theme"=FALSE} ("Set App Theme Argument"), Variant=w656) -> (data=w654:T22, error out=w659:errorcluster)
            n109 = Unbundle By Name(w654) -> ("Theme"=w651:bool)
            n110 = control-ref of="This VI"() -> (w653:refnum<vi>)
            n111 = Bundle By Name(cluster=w657, "Theme"=w651) -> (w652:T5)
            n112 = call "Set Theme.vi"("Dark?"=w651, "VI in"=w653) -> ()  [unwired: 10 in]
            n113 = call "Theme Updated.vi"("Theme"=w651) -> ()  [unwired: 10 in, 1 out]
            n114 = call "Save Theme in config.vi"("error in"=w659, "Theme"=w651) -> ("error out"=w660:errorcluster)  [unwired: 9 in]
            n115 = call "Register controls Mouse Enter.vi"("error in"=w660) -> ("error out"=w658:errorcluster)  [unwired: 10 in]
          }
          frame "Show About" {
            # "Show About project"
            n116 = Variant To Data(error in=w670, type=T23 {"Boolean"=FALSE} ("Show About Argument"), Variant=w664) -> (error out=w667:errorcluster)  [unwired: 1 out]
            n117 = control-ref of="This VI"() -> (w662:refnum<vi>)
            n118 = call "Hide VI Panel.vi"("error in (no error)"=w667, "VI"=w662) -> ("error out"=w669:errorcluster)  [unwired: 9 in]
            n119 = call "About Panther Dashboard.vi"("error in"=w669) -> ("error out"=w668:errorcluster)  [unwired: 10 in]
            n120 = call "Open VI Panel.vi"("error in (no error)"=w668, "VI"=w662) -> ("error out"=w666:errorcluster)  [unwired: 9 in]
          }
          frame "Update Module ID" {
            # "Update the Current Module ID"
            n121 = Variant To Data(error in=w678, type=T24 {"New ID"=-1} ("Update Module ID Argument"), Variant=w675) -> (data=w673:T24, error out=w677:errorcluster)
            n122 = Unbundle By Name(w673) -> ("New ID"=w671:i32)
            n123 = Bundle By Name(cluster=w676, "Module ID"=w671) -> (w672:T5)
          }
          frame "Save Library Description" {
            # "Save Library Description"
            n124 = Variant To Data(error in=w688, type=T25 {"Library Description"=""} ("Save Library Description Argument"), Variant=w684) -> (data=w682:T25, error out=w687:errorcluster)
            n125 = Unbundle By Name(w682) -> ("Library Description"=w681:string)
            n126 = in-place {
              in-place-border: w681 -> [w692]
              in-place-border: [w694] -> w685
              n127 = in-place-cluster #1(w680) -> ("Current Selection.DQMH Lib Ref"=w693:refnum<vi>, "DQMH Scan Results"=w690:T8)
              n128 = call "Save Library Documentation.vi"("New Description"=w692, "DQMH Modules Info In"=w690, "Library in"=w693) -> ("error out"=w694:errorcluster, "DQMH Modules Info Out"=w691:T8, "Lib out"=w689:refnum<vi>)  [unwired: 6 in]
              n129 = in-place-cluster #1("Current Selection.DQMH Lib Ref"=w689, "DQMH Scan Results"=w691) -> (w679:T5)
            }
            n130 = Merge Errors(w687, w685) -> (w686:errorcluster)
          }
          frame "Save VI Description" {
            # "Save Event Description"
            n131 = Variant To Data(error in=w704, type=T26 {"VI Description"=""} ("Save VI Description Argument"), Variant=w700) -> (data=w698:T26, error out=w703:errorcluster)
            n132 = Unbundle By Name(w698) -> ("VI Description"=w696:string)
            n133 = in-place {
              in-place-border: w696 -> [w707]
              in-place-border: [w708] -> w701
              n134 = in-place-cluster #2(w697) -> ("Current Selection.VI Ref"=w706:refnum<vi>)
              n135 = call "Save Event Description.vi"("Event Description"=w707, "Event Ref in"=w706) -> ("error out"=w708:errorcluster, "Event Ref out"=w705:refnum<vi>)  [unwired: 8 in]
              n136 = in-place-cluster #2("Current Selection.VI Ref"=w705) -> (w695:T5)
            }
            n137 = Merge Errors(w703, w701) -> (w702:errorcluster)
          }
          frame "Save Project Documentation" {
            n138 = Variant To Data(error in=w717, type=T28 {"Project Description"=""} ("Save Project Documentation Argument"), Variant=w714) -> (data=w712:T28, error out=w716:errorcluster)
            n139 = Unbundle By Name(w712) -> ("Project Description"=w709:string)
            n140 = Unbundle By Name(w711) -> ("DQMH Scan Results.Project References.Project Ref"=w710:refnum<vi>)
            n141 = property class="Project"(reference=w710, error in=w716, "Description"=w709) -> (error out=w715:errorcluster)  [unwired: 1 out]
          }
          frame "---Copy This Frame---" {
            # "Duplicate this frame when creating new messages.  Change this comment in the duplicated frame to describe this message."
            n142 = Merge Errors(w720) -> (w719:errorcluster)
          }
          frame "---Exit and Error Handling---" {
            # "Separator - The following cases handle errors and exit messages."
          }
          frame "Error" {
            # "Error - Check the error message data and respond accordingly. This message is sent by the \"Error Handler\" VIs at the end of each loop in this application."
            n143 = property on="Property Node" class="Module Admin"(reference=w724) -> ("Accessors:External Launch"=w723:bool)  [unwired: 1 in, 2 out]
            n144 = Variant To Data(error in=w732, type=errorcluster {"status"=FALSE, "code"=0, "source"=""} ("error constant"), Variant=w726) -> (data=w733:errorcluster, error out=w730:errorcluster)
            n145 = call "Error Reported.vi"("Error"=w733) -> ()  [unwired: 10 in, 1 out]
            n146 = case shown="True" w723 {
              tunnel: [w738 _] -> w729
              tunnel: w725 -> [w736 _]
              tunnel: w733 -> [w737 _]
              frame False {
                # "If the module is running standalone, then pop up an error dialog and call the \"Exit\" message."
                n147 = call <vilib>:"Simple Error Handler.vi"("error in (no error)"=w737) -> ()  [unwired: 4 in, 5 out]
                n148 = call-poly <vilib>:"Delacor_lib_QMH_Enqueue Message (poly).vi"("Priority Message? (F)"=TRUE, "Message"="Exit", "Message Queue in"=w736) -> ("error out"=w738:errorcluster)  [unwired: 7 in, 1 out]
              }
              frame True {
                # "If the module was launched externally, calling the Error Reported broadcast VI is the only action performed by the \"Error\" message. The module's caller can then process the error appropriately."
              }
            }
            n149 = Merge Errors(w730, w729) -> (w728:errorcluster)
            n150 = local write "error out"(w728) -> ()
          }
          frame "Exit" {
            w745 = 91  # 91: not all Exit messages will have an argument
            w747 = TRUE  # Stop the VI
            # "Release the message queue reference"
            # "Exit - Exit the application."
            n151 = Variant To Data(error in=w754, type=T20 {"Origin"="", "Exit via Stop Module Req?"=FALSE, "Wait for Module to stop?"=FALSE} ("Stop Argument"), Variant=w746) -> (data=w743:T20, error out=w750:errorcluster)
            n152 = call <vilib>:"Clear Errors.vi"("error in (no error)"=w750, "specific error code to clear (0: all)"=w745) -> ("error out"=w753:errorcluster)  [unwired: 4 in, 1 out]
            n153 = control-ref of="This VI"() -> (w742:refnum<vi>)
            n154 = invoke on="Modules Tree" class="Tree (strict)" method="Edit Tree Items.Delete"() -> ()  [unwired: 5 in, 5 out]
            n155 = call-dynamic "Delacor_lib_QMH_Release Message Queue.vi"("error in"=w753, "Message Queue"=w748) -> ("error out"=w752:errorcluster)  [unwired: 9 in]
            n156 = call "Handle Exit.vi"("Stop Argument"=w743, "Admin in"=w741, "VI reference"=w742) -> ("error out"=w749:errorcluster)  [unwired: 7 in, 1 out]
            n157 = call "Close vi references.vi"("Data Cluster"=w740) -> ()  [unwired: 10 in, 1 out]
            n158 = Merge Errors(w752, w749) -> (w751:errorcluster)
            n159 = call "Stop Module.vi"("Origin"="Panther Dahsboard Stopped") -> ()  [unwired: 10 in, 1 out]
          }
          frame Default {
            # "'Default' case only runs if there is a message that isn't defined in any of the other cases.  Output a programming error."
            n160 = call "Module Name--constant.vi"() -> ("Module Name"=w755:string)  [unwired: 11 in]
            n161 = xnode ("Error Ring")("parameter 0"=w756, "parameter 1"=w755) -> ("error out"=w760:errorcluster)
            n162 = Merge Errors(w758, w760) -> (w759:errorcluster)
          }
        }
        n163 = call-dynamic "Delacor_lib_QMH_Error Handler - Message Handling Loop.vi"("error in"=w437, "Ignore Errors (Runtime)"=w425, "Message Queue in"=w427) -> ("dup error in"=w434:errorcluster)  [unwired: 7 in, 1 out]
      }
      n164 = while {
        tunnel: w30 -> [w139]
        shift-right: [w141] -> w36
        shift-left: w34 -> [w142]
        tunnel: [w143] -> w39
        shift-right: [w137] -> _
        shift-left: w29 -> [w136]
        shift-right: [w135] -> _
        shift-left: Selection_Type--enum."Public API" ("Selection type") -> [w134]
        stop <- w140 stop-if-true
        # "Event Handling Loop"
        n165 = event "DQMH_EVENT_MAIN" shown="[33] <Panther Dashboard Request Events.Save Project Documentation>: User Event" {
          selector: w142 -> [_ _ _ _ _ _ _ _ _ _ _ _ _ _ _ _ _ _ _ _ _ _ _ _ _ _ _ _ _ _ _ _ _ _]
          dyn-events: [_ _ _ _ _ _ _ _ _ _ _ _ _ _ _ _ _ _ _ _ _ _ _ _ _ _ _ _ _ _ _ _ _ _] -> w141
          timeout: 3000 -> [_ _ _ _ _ _ _ _ _ _ _ _ _ _ _ _ _ _ _ _ _ _ _ _ _ _ _ _ _ _ _ _ _ _]
          tunnel: [_ _ _ _ _ _ _ _ _ _ _ _ _ _ _ _ _ _ _ TRUE ("Discard?") _ _ _ _ _ _ _ _ _ _ _ _ _ _] -> w140
          tunnel: w139 -> [w145 _ _ w180 w185 w197 w202 w221 _ w230 _ w244 w254 _ _ w271 w280 _ _ w313 w322 _ w333 w341 w349 w357 w365 w373 w381 w389 w397 w405 w413 w421]
          tunnel: [w154 w168 w173 w181 w186 w198 w203 w222 w227 w233 w241 w247 w255 w259 _ w272 w281 _ _ w316 w324 w328 w336 w344 w352 w360 w368 w376 w384 w392 w400 w408 w416 w424] -> w144
          tunnel: [w153 w167 w172 w175 w183 w194 w200 w217 w223 w232 w240 w246 w249 w257 w261 w265 w278 w293 w304 w306 w319 w327 w335 w343 w351 w359 w367 w375 w383 w391 w399 w407 w415 w423] -> w137
          tunnel: w136 -> [w153 w167 w172 w175 w183 w194 w200 _ w223 w232 w240 w246 w249 w257 w261 w265 w278 w293 w304 w306 w319 w327 w335 w343 w351 w359 w367 w375 w383 w391 w399 w407 w415 w423]
          tunnel: [w152 w166 w171 w174 w182 w193 w199 w215 w225 w231 w239 w245 w248 w256 w260 w264 w277 w292 w303 w305 w318 w326 w334 w342 w350 w358 w366 w374 w382 w390 w398 w406 w414 w422] -> w135
          tunnel: w134 -> [w152 w166 w171 w174 _ w193 w199 _ w225 w231 w239 w245 w248 w256 w260 w264 w277 w292 w303 w305 w318 w326 w334 w342 w350 w358 w366 w374 w382 w390 w398 w406 w414 w422]
          event "Add Event", "Remove Event", "Convert Event", "Rename Event", "Add New Module", "Rename Module", "Validate Module", "Create Module Template", "Add Unit Test Module", "Create RT Tester Module": Value Change {
            n166 = event-data() -> ("CtlRef"=w150:refnum<vi>)  [unwired: 1 in]
            n167 = property class="Bool"(reference=w150) -> ("Label.Text"=w151:string)  [unwired: 1 in, 2 out]
            n168 = case shown="\"Create Module Template\"" w151 {
              tunnel: [DQMH_Tools_Menu--enum."Create New DQMH Event" ("DQMH Tools") DQMH_Tools_Menu--enum."Convert DQMH Event" ("DQMH Tools") DQMH_Tools_Menu--enum."Remove DQMH Event" ("DQMH Tools") DQMH_Tools_Menu--enum."Rename DQMH Event" ("DQMH Tools") DQMH_Tools_Menu--enum."Add New DQMH Module" ("DQMH Tools") DQMH_Tools_Menu--enum."Rename DQMH Module" ("DQMH Tools") DQMH_Tools_Menu--enum."Validate DQMH Module" ("DQMH Tools") DQMH_Tools_Menu--enum."Create RT Tester" ("DQMH Tools") DQMH_Tools_Menu--enum."New DQMH  Unit Test" ("DQMH Tools") DQMH_Tools_Menu--enum."Create DQMH Module Template" ("DQMH Tools")] -> w146
              frame "Add Event", Default {
              }
              frame "Convert Event" {
              }
              frame "Remove Event" {
              }
              frame "Rename Event" {
              }
              frame "Add New Module" {
              }
              frame "Rename Module" {
              }
              frame "Validate Module" {
              }
              frame "Create RT Tester Module" {
              }
              frame "Add Unit Test Module" {
              }
              frame "Create Module Template" {
              }
            }
            n169 = Bundle(cluster=T13 {"Scripting Tool"=enum."Create New DQMH Event"} ("Launch DQMH Scripting Tools Argument"), "Scripting Tool"=w146) -> (w149:T13)
            n170 = call-poly <vilib>:"Delacor_lib_QMH_Enqueue Message (poly).vi"("Message Data"=w149, "Message"="Launch DQMH Scripting Tools", "Message Queue in"=w145) -> ("error out"=w154:errorcluster)  [unwired: 7 in, 1 out]
          }
          event "Context Help Panther": Value Change {
            # "Open Documentation DQMH Module"
            n171 = event-data() -> ()  [unwired: 1 in, 1 out]
            n172 = case shown="True" "Context Help Panther" {
              tunnel: [w169 w170] -> w168
              frame False {
                n173 = call "Hide Panel.vi"() -> ("error out"=w169:errorcluster)  [unwired: 11 in]
              }
              frame True {
                n174 = call "Show Panel.vi"() -> ("error out"=w170:errorcluster)  [unwired: 11 in]
              }
            }
          }
          event User Event {
            # "We wait for the Context help module to init to request to refresh \npanther Dashboard Broadcasts, we need this module to be\nlistening Panther Dashboard broadcasts"
            n175 = event-data() -> ()  [unwired: 1 in, 1 out]
            n176 = call "Refresh Panther Dashboard Broadcasts.vi"() -> ("error out"=w173:errorcluster)  [unwired: 11 in]
          }
          event "Expand Results": Value Change {
            # "Expand or close Result tree"
            n177 = event-data() -> ()  [unwired: 1 in, 1 out]
            n178 = Bundle(cluster=T15 {"Expand?"=FALSE} ("Expand or Close Argument"), "Expand?"="Expand Results") -> (w177:T15)
            n179 = call-poly <vilib>:"Delacor_lib_QMH_Enqueue Message (poly).vi"("Message Data"=w177, "Message"="Expand or Close", "Message Queue in"=w180) -> ("error out"=w181:errorcluster)  [unwired: 7 in, 1 out]
          }
          event "Modules Tree": Double Click {
            # "User double click an element on the tree control, we check if it is an event to find its frame on the corresponding DQMH module, we also check if it is a broadcast to find where is being triggered"
            n180 = event-data() -> ("Tag"=w184:string)  [unwired: 1 in]
            n181 = call "Validate if event is selected.vi"("Tree Selection"=w184) -> ("Selection type"=w182:T4)  [unwired: 10 in]
            n182 = case shown="\"Module\"" w182 {
              tunnel: [w189 _ w192] -> w186
              tunnel: w185 -> [w188 _ w191]
              frame "Module" {
                # "Selection is a module"
                n183 = call-poly <vilib>:"Delacor_lib_QMH_Enqueue Message (poly).vi"("Message"="Find Module in project", "Message Queue in"=w188) -> ("error out"=w189:errorcluster)  [unwired: 8 in, 1 out]
              }
              frame "Public API" {
              }
              frame "Broadcast", "Request" {
                # "Selection is an Event vi?"
                n184 = call-poly <vilib>:"Delacor_lib_QMH_Enqueue Message (poly).vi"("Message"="Locate Event on Main", "Message Queue in"=w191) -> ("error out"=w192:errorcluster)  [unwired: 8 in, 1 out]
              }
            }
          }
          event "Modules Tree": Drag Starting? {
            # "Drag current selection to user destination"
            n185 = event-data() -> ()  [unwired: 1 in, 1 out]
            n186 = call-poly <vilib>:"Delacor_lib_QMH_Enqueue Message (poly).vi"("Message"="Drag VI", "Message Queue in"=w197) -> ("error out"=w198:errorcluster)  [unwired: 8 in, 1 out]
            n187 = event-data("Discard?"=TRUE) -> ()  [unwired: 1 in, 1 out]
          }
          event "Modules Tree": Shortcut Menu Selection (User) {
            # "User selects something from the Right Click Shortcut Menu"
            n188 = event-data() -> ("ItemTag"=w201:string)  [unwired: 1 in]
            n189 = case shown="Default" w201 {
              selector: w201 -> [w206 w212]
              tunnel: w202 -> [w210 w213]
              tunnel: [w211 w214] -> w203
              frame "-Run: Hide Panel", "-Run: Show Diagram", "-Run: Show Panel", "-Run: Stop Module" {
                n190 = Match Pattern(string=w206, regular expression="-Run: ") -> (after substring=w205:string)  [unwired: 1 in, 3 out]
                n191 = Bundle(cluster=T16 {"Event Name"=""} ("Execute Default Event Request Argument"), "Event Name"=w205) -> (w208:T16)
                n192 = call-poly <vilib>:"Delacor_lib_QMH_Enqueue Message (poly).vi"("Message Data"=w208, "Message"="Execute Default Event Request", "Message Queue in"=w210) -> ("error out"=w211:errorcluster)  [unwired: 7 in, 1 out]
              }
              frame Default {
                n193 = call-poly <vilib>:"Delacor_lib_QMH_Enqueue Message (poly).vi"("Message"=w212, "Message Queue in"=w213) -> ("error out"=w214:errorcluster)  [unwired: 8 in, 1 out]
              }
            }
          }
          event "Modules Tree": Value Change {
            w217 = TRUE  # Tree valid Selection
            # "The user selected an item on the tree control"
            n194 = event-data() -> ()  [unwired: 1 in, 1 out]
            n195 = Bundle(cluster=T17 {"Tree DQMH Sel"=""} ("Tree DQMH Selection Argument"), "Tree DQMH Sel"="Modules Tree") -> (w218:T17)
            n196 = call "Validate if event is selected.vi"("Tree Selection"="Modules Tree") -> ("Selection type"=w215:T4)  [unwired: 10 in]
            n197 = call-poly <vilib>:"Delacor_lib_QMH_Enqueue Message (poly).vi"("Message Data"=w218, "Message"="Tree DQMH Selection", "Message Queue in"=w221) -> ("error out"=w222:errorcluster)  [unwired: 7 in, 1 out]
          }
          event "Modules Tree": Shortcut Menu Activation? {
            # "This is wher the shorcut menu is filled, only after the user select a module"
            n198 = event-data() -> ("MenuRef"=w226:refnum<k9>)  [unwired: 1 in]
            n199 = call "Create Tree Shortcut Menu.vi"("Selection type"=w225, "Menu in"=w226) -> ("error out"=w227:errorcluster)  [unwired: 9 in]
            n200 = Not(x=w223) -> (.not. x?=w224:bool)
            n201 = event-data("Discard?"=w224) -> ()  [unwired: 1 in, 1 out]
          }
          event "Projects": Value Change {
            n202 = event-data() -> ()  [unwired: 1 in, 1 out]
            n203 = call-poly <vilib>:"Delacor_lib_QMH_Enqueue Message (poly).vi"("Message Data"="Projects", "Message"="Refresh Targets", "Message Queue in"=w230) -> ("error out"=w233:errorcluster)  [unwired: 7 in, 1 out]
          }
          event "Projects": Shortcut Menu Activation? {
            n204 = event-data() -> ("MenuRef"=w238:refnum<k9>)  [unwired: 1 in]
            n205 = Delete Menu Items(9:w238) -> (0:w242:errorcluster, 3:w237:refnum<k9>)  [unwired: 3 in]
            n206 = Insert Menu Items(6:w242, 8:string[] ["Open Project Folder"] ("item names"), 9:w237) -> (0:w241:errorcluster)  [unwired: 3 in, 2 out]
            n207 = local read "Projects"() -> (w235:string)
            n208 = Empty String/Path?(string/path=w235) -> (empty?=w234:bool)
            n209 = event-data("Discard?"=w234) -> ()  [unwired: 1 in, 1 out]
          }
          event "Projects": Shortcut Menu Selection (User) {
            n210 = event-data() -> ("ItemTag"=w243:string)  [unwired: 1 in]
            n211 = call-poly <vilib>:"Delacor_lib_QMH_Enqueue Message (poly).vi"("Message"=w243, "Message Queue in"=w244) -> ("error out"=w247:errorcluster)  [unwired: 8 in, 1 out]
          }
          event User Event {
            # "Another Module called the \"Expand or Close\" API Method."
            n212 = event-data() -> ("Expand?"=w250:bool)  [unwired: 1 in]
            n213 = Bundle(cluster=T15 {"Expand?"=FALSE} ("Expand or Close Argument"), "Expand?"=w250) -> (w251:T15)
            n214 = call-poly <vilib>:"Delacor_lib_QMH_Enqueue Message (poly).vi"("Message Data"=w251, "Message"="Expand or Close", "Message Queue in"=w254) -> ("error out"=w255:errorcluster)  [unwired: 7 in, 1 out]
          }
          event User Event {
            # "Another Module called the \"Get Module Execution Status\" API Method."
            n215 = event-data() -> ()  [unwired: 1 in, 1 out]
            n216 = call "Update Module Execution Status.vi"("Running?"=TRUE) -> ("error out"=w259:errorcluster)  [unwired: 10 in]
          }
          event User Event {
            # "Hide the panel of this VI, and send a status updated message to let listeners know."
            # "Another Module called the \"Hide Panel\" API Method."
            n217 = event-data() -> ()  [unwired: 1 in, 1 out]
            n218 = control-ref of="This VI"() -> (w262:refnum<vi>)
            n219 = call "Hide VI Panel.vi"("VI"=w262) -> ()  [unwired: 10 in, 1 out]
          }
          event User Event {
            # "Another Module called the \"Scan DQMH Modules\" API Method."
            n220 = event-data() -> ("Include Dependencies"=w267:bool, "Project"=w266:string, "Target"=w263:string)  [unwired: 1 in]
            n221 = Bundle(cluster=T18 {"Include Dependencies"=FALSE, "Project"="", "Target"=""} ("Scan DQMH Modules Argument"), "Include Dependencies"=w267, "Project"=w266, "Target"=w263) -> (w268:T18)
            n222 = call-poly <vilib>:"Delacor_lib_QMH_Enqueue Message (poly).vi"("Message Data"=w268, "Message"="Scan DQMH Modules", "Message Queue in"=w271) -> ("error out"=w272:errorcluster)  [unwired: 7 in, 1 out]
          }
          event "Search": Value Change {
            # "#via_ignore Unwired Event Nodes"
            # "Another Module called the \"Scan DQMH Modules\" API Method."
            n223 = event-data() -> ()  [unwired: 1 in, 1 out]
            n224 = local read "Projects"() -> (w276:string)
            n225 = Empty String/Path?(string/path="Targets") -> (empty?=w274:bool)
            n226 = global write "Panther Dashboard--global.vi" "Target"("Targets") -> ()
            n227 = Empty String/Path?(string/path=w276) -> (empty?=w279:bool)
            n228 = Or(x=w279, y=w274) -> (x .or. y?=w275:bool)
            n229 = case shown="False" w275 {
              tunnel: [w289 _] -> w281
              tunnel: w280 -> [w288 _]
              tunnel: w276 -> [w283 _]
              tunnel: "Targets" -> [w282 _]
              frame False {
                n230 = Bundle(cluster=T18 {"Include Dependencies"=FALSE, "Project"="", "Target"=""} ("Scan DQMH Modules Argument"), "Include Dependencies"="Include Dependencies", "Project"=w283, "Target"=w282) -> (w285:T18)
                n231 = call-poly <vilib>:"Delacor_lib_QMH_Enqueue Message (poly).vi"("Message Data"=w285, "Message"="Scan DQMH Modules", "Message Queue in"=w288) -> ("error out"=w289:errorcluster)  [unwired: 7 in, 1 out]
              }
              frame True {
                n232 = invoke on="Projects" class="CmbBox" method="ObjHighlight"() -> (error out=w291:errorcluster)  [unwired: 3 in, 2 out]
                n233 = invoke on="Targets" class="CmbBox" method="ObjHighlight"(error in=w291) -> ()  [unwired: 2 in, 3 out]
                n234 = call "Status Updated.vi"("Status"="Scanning requires a project and an target please make the selection.\n") -> ()  [unwired: 10 in, 1 out]
              }
            }
          }
          event User Event {
            # "Another Module called the \"Show Diagram\" API Method. This event is used for debugging."
            n235 = event-data() -> ()  [unwired: 1 in, 1 out]
            n236 = disable-structure shown="RUN_TIME_ENGINE==False" {
              frame condition #0 (active) {
                # "functionality not available in exe"
                n237 = invoke on="Invoke Node" class="VI" method="Lock State.Get"() -> (error out=w299:errorcluster, "Get Lock State"=w298:T19, "pwd in cache"=w295:bool)  [unwired: 4 in, 1 out]
                n238 = Equal?(x=T19."Password-protected", y=w298) -> (x = y?=w296:bool)
                n239 = Compound Arithmetic op=AND(w296, invert w295) -> (w294:bool)
                n240 = case shown="False" w294 {
                  tunnel: w299 -> [w301 _]
                  frame False {
                    n241 = property on="Property Node" class="VI"(error in=w301, "BDWin.Open"=TRUE ("Block Diagram Window:Open")) -> ()  [unwired: 1 in, 2 out]
                  }
                  frame True {
                    # "Password-protected VI, and the password is not in the cache. Do not show the diagram."
                  }
                }
              }
              frame condition #1 {
              }
            }
          }
          event User Event {
            # "Show the panel of this VI, and send a status updated message to let listeners know."
            # "Another Module called the \"Show Panel\" API Method."
            n242 = event-data() -> ()  [unwired: 1 in, 1 out]
            n243 = control-ref of="This VI"() -> (w302:refnum<vi>)
            n244 = call "Open VI Panel.vi"("VI"=w302) -> ()  [unwired: 10 in, 1 out]
          }
          event User Event {
            # "The Stop Module Event can get fired from the Exit message in the MHL. The queue gets destroyed in that case. If the queue no longer exists, the Enqueue Exit as a priority message will return error 1. It is safe to ignore, because the module is already exiting."
            # "Another Module called the \"Stop Module\" API Method  or the Message Handling Loop below."
            n245 = event-data() -> ("Exit via Stop Module Req?"=w309:bool, "Wait for Module to stop?"=w308:bool)  [unwired: 1 in]
            n246 = Bundle By Name(cluster=T20 {"Origin"="", "Exit via Stop Module Req?"=FALSE, "Wait for Module to stop?"=FALSE} ("Stop Argument"), "Exit via Stop Module Req?"=w309, "Wait for Module to stop?"=w308) -> (w307:T20)
            n247 = call-poly <vilib>:"Delacor_lib_QMH_Enqueue Message (poly).vi"("Priority Message? (F)"=TRUE, "Message Data"=w307, "Message"="Exit", "Message Queue in"=w313) -> ("error out"=w317:errorcluster)  [unwired: 6 in, 1 out]
            n248 = call <vilib>:"Clear Errors.vi"("error in (no error)"=w317, "specific error code to clear (0: all)"=1) -> ("error out"=w316:errorcluster)  [unwired: 4 in, 1 out]
          }
          event Panel Close? {
            w323 = TRUE  # Discard the event, the MHL is responsible for closing and stopping this VI.
            # "Hide the panel or send the 'Exit' message if the user clicks the 'X' on the module main VI panel."
            n249 = event-data() -> ()  [unwired: 1 in, 1 out]
            n250 = call-poly <vilib>:"Delacor_lib_QMH_Enqueue Message (poly).vi"("Priority Message? (F)"=TRUE, "Message"="Exit", "Message Queue in"=w322) -> ("error out"=w324:errorcluster)  [unwired: 7 in, 1 out]
            n251 = event-data ("Event Filter Node")("Discard?"=w323) -> ()  [unwired: 1 in, 1 out]
          }
          event Timeout {
            w325 = FALSE  # Init?
            n252 = event-data() -> ()  [unwired: 1 in, 1 out]
            n253 = call "Scan For App Projects.vi"("Init?"=w325) -> ("error out"=w328:errorcluster)  [unwired: 10 in]
          }
          event User Event {
            # "Another Module called the \"Launch DQMH Scripting Tools\" API Method."
            n254 = event-data() -> ("Scripting Tool"=w329:T14)  [unwired: 1 in]
            n255 = Bundle(cluster=T13 {"Scripting Tool"=enum."Create New DQMH Event"} ("Launch DQMH Scripting Tools Argument"), "Scripting Tool"=w329) -> (w330:T13)
            n256 = call-poly <vilib>:"Delacor_lib_QMH_Enqueue Message (poly).vi"("Message Data"=w330, "Message"="Launch DQMH Scripting Tools", "Message Queue in"=w333) -> ("error out"=w336:errorcluster)  [unwired: 7 in, 1 out]
          }
          event User Event {
            # "Another Module called the \"Generate Project Documentation\" API Method."
            n257 = event-data() -> ("Boolean"=w337:bool)  [unwired: 1 in]
            n258 = Bundle(cluster=T21 {"Boolean"=FALSE} ("Generate Project Documentation Argument"), "Boolean"=w337) -> (w338:T21)
            n259 = call-poly <vilib>:"Delacor_lib_QMH_Enqueue Message (poly).vi"("Message Data"=w338, "Message"="Generate Project Documentation", "Message Queue in"=w341) -> ("error out"=w344:errorcluster)  [unwired: 7 in, 1 out]
          }
          event User Event {
            # "Another Module called the \"Set App Theme\" API Method."
            n260 = event-data() -> ("Theme"=w345:bool)  [unwired: 1 in]
            n261 = Bundle(cluster=T22 {"Theme"=FALSE} ("Set App Theme Argument"), "Theme"=w345) -> (w346:T22)
            n262 = call-poly <vilib>:"Delacor_lib_QMH_Enqueue Message (poly).vi"("Message Data"=w346, "Message"="Set App Theme", "Message Queue in"=w349) -> ("error out"=w352:errorcluster)  [unwired: 7 in, 1 out]
          }
          event "Theme Panther": Value Change {
            # "Another Module called the \"Set App Theme\" API Method."
            n263 = event-data() -> ()  [unwired: 1 in, 1 out]
            n264 = Bundle(cluster=T22 {"Theme"=FALSE} ("Set App Theme Argument"), "Theme"="Theme Panther") -> (w354:T22)
            n265 = call-poly <vilib>:"Delacor_lib_QMH_Enqueue Message (poly).vi"("Message Data"=w354, "Message"="Set App Theme", "Message Queue in"=w357) -> ("error out"=w360:errorcluster)  [unwired: 7 in, 1 out]
          }
          event User Event {
            # "Another Module called the \"Show About\" API Method."
            n266 = event-data() -> ("Boolean"=w361:bool)  [unwired: 1 in]
            n267 = Bundle(cluster=T23 {"Boolean"=FALSE} ("Show About Argument"), "Boolean"=w361) -> (w362:T23)
            n268 = call-poly <vilib>:"Delacor_lib_QMH_Enqueue Message (poly).vi"("Message Data"=w362, "Message"="Show About", "Message Queue in"=w365) -> ("error out"=w368:errorcluster)  [unwired: 7 in, 1 out]
          }
          event "About Panther": Value Change {
            # "Another Module called the \"Show About\" API Method."
            n269 = event-data() -> ()  [unwired: 1 in, 1 out]
            n270 = Bundle(cluster=T23 {"Boolean"=FALSE} ("Show About Argument"), "Boolean"="About Panther") -> (w370:T23)
            n271 = call-poly <vilib>:"Delacor_lib_QMH_Enqueue Message (poly).vi"("Message Data"=w370, "Message"="Show About", "Message Queue in"=w373) -> ("error out"=w376:errorcluster)  [unwired: 7 in, 1 out]
          }
          event User Event {
            # "Another Module called the \"Update Module ID\" API Method."
            n272 = event-data() -> ("New ID"=w377:i32)  [unwired: 1 in]
            n273 = Bundle(cluster=T24 {"New ID"=-1} ("Update Module ID Argument"), "New ID"=w377) -> (w378:T24)
            n274 = call-poly <vilib>:"Delacor_lib_QMH_Enqueue Message (poly).vi"("Message Data"=w378, "Message"="Update Module ID", "Message Queue in"=w381) -> ("error out"=w384:errorcluster)  [unwired: 7 in, 1 out]
          }
          event "Module ID": Value Change {
            # "Another Module called the \"Update Module ID\" API Method."
            n275 = event-data() -> ()  [unwired: 1 in, 1 out]
            n276 = Bundle(cluster=T24 {"New ID"=-1} ("Update Module ID Argument"), "New ID"="Module ID") -> (w386:T24)
            n277 = call-poly <vilib>:"Delacor_lib_QMH_Enqueue Message (poly).vi"("Message Data"=w386, "Message"="Update Module ID", "Message Queue in"=w389) -> ("error out"=w392:errorcluster)  [unwired: 7 in, 1 out]
          }
          event User Event {
            # "Another Module called the \"Save Library Description\" API Method."
            n278 = event-data() -> ("Library Description"=w393:string)  [unwired: 1 in]
            n279 = Bundle(cluster=T25 {"Library Description"=""} ("Save Library Description Argument"), "Library Description"=w393) -> (w394:T25)
            n280 = call-poly <vilib>:"Delacor_lib_QMH_Enqueue Message (poly).vi"("Message Data"=w394, "Message"="Save Library Description", "Message Queue in"=w397) -> ("error out"=w400:errorcluster)  [unwired: 7 in, 1 out]
          }
          event User Event {
            # "Another Module called the \"Save VI Description\" API Method."
            n281 = event-data() -> ("VI Description"=w401:string)  [unwired: 1 in]
            n282 = Bundle(cluster=T26 {"VI Description"=""} ("Save VI Description Argument"), "VI Description"=w401) -> (w402:T26)
            n283 = call-poly <vilib>:"Delacor_lib_QMH_Enqueue Message (poly).vi"("Message Data"=w402, "Message"="Save VI Description", "Message Queue in"=w405) -> ("error out"=w408:errorcluster)  [unwired: 7 in, 1 out]
          }
          event User Event {
            # "Another Module called the \"Open Documentation\" API Method."
            n284 = event-data() -> ("Boolean"=w409:bool)  [unwired: 1 in]
            n285 = Bundle(cluster=T27 {"Boolean"=FALSE} ("Open Documentation Argument"), "Boolean"=w409) -> (w410:T27)
            n286 = call-poly <vilib>:"Delacor_lib_QMH_Enqueue Message (poly).vi"("Message Data"=w410, "Message"="Open Documentation", "Message Queue in"=w413) -> ("error out"=w416:errorcluster)  [unwired: 7 in, 1 out]
          }
          event User Event {
            # "Another Module called the \"Save Project Documentation\" API Method."
            n287 = event-data() -> ("Project Description"=w417:string)  [unwired: 1 in]
            n288 = Bundle(cluster=T28 {"Project Description"=""} ("Save Project Documentation Argument"), "Project Description"=w417) -> (w418:T28)
            n289 = call-poly <vilib>:"Delacor_lib_QMH_Enqueue Message (poly).vi"("Message Data"=w418, "Message"="Save Project Documentation", "Message Queue in"=w421) -> ("error out"=w424:errorcluster)  [unwired: 7 in, 1 out]
          }
        }
        n290 = call-dynamic "Delacor_lib_QMH_Error Handler - Event Handling Loop.vi"("error in"=w144, "Message Queue in"=w139) -> ("dup error in"=w143:errorcluster)  [unwired: 8 in, 1 out]
      }
      n291 = while {
        tunnel: w33 -> [w50]
        tunnel: [w49] -> w32
        shift-right: [w47] -> _
        shift-left: -1 -> [w46]
        shift-right: [w45] -> _
        shift-left: _ -> [w44]
        tunnel: w30 -> [w43]
        tunnel: [w51] -> w37
        shift-right: [w42] -> _
        shift-left: _ -> [w41]
        stop <- w48 stop-if-true
        # "Helper Loop"
        n292 = event shown="[6] <event source>: Mouse Enter" {
          selector: w50 -> [_ _ _ _ _ _ _ w111 _ _ _]
          dyn-events: [_ _ _ _ _ _ _ w109 _ _ _] -> w49
          timeout: w46 -> [_ _ _ _ _ _ _ _ _ _ _]
          tunnel: [_ TRUE _ _ _ _ _ _ _ _ _] -> w48
          tunnel: [w54 w59 w64 w77 w89 w93 w104 w110 w118 w129 w133] -> w45
          tunnel: [w55 w60 500 w76 w88 w92 w103 w113 w117 w128 w132] -> w47
          tunnel: w46 -> [w55 w60 _ w76 w88 w92 w103 w113 w117 w128 w132]
          tunnel: w44 -> [w54 w59 _ w77 w89 w93 w104 w110 w118 w129 w133]
          tunnel: [w56 _ _ _ _ _ _ _ w119 _ _] -> w52
          tunnel: [w53 w57 w62 w75 w86 w91 w102 w112 w116 w127 w131] -> w42
          tunnel: w41 -> [w53 w57 _ w75 w86 w91 w102 w112 w116 w127 w131]
          event Timeout {
            n293 = event-data() -> ()  [unwired: 1 in, 1 out]
            n294 = call "Get Module Execution Status by ref.vi"("Modules Tree ref"=w53, "Refs"=w54) -> ("error out"=w56:errorcluster)  [unwired: 9 in]
          }
          event User Event {
            n295 = event-data() -> ()  [unwired: 1 in, 1 out]
            n296 = Unbundle By Name(w59) -> ("Modules"=w58:refnum<vi>[])
            n297 = Close Reference(reference=w58) -> ()  [unwired: 1 in, 1 out]
          }
          event User Event {
            # "Refresh time"
            n298 = event-data() -> ("Modules"=w67:refnum<vi>[], "Modules Types"=w65:T9[], "Application Instance"=w66:refnum<vi>)  [unwired: 1 in]
            n299 = Bundle By Name(cluster=T11 {"Modules"=[], "Modules Types"=[], "Application Instance"=refnum}, "Modules"=w67, "Modules Types"=w65, "Application Instance"=w66) -> (w64:T11)
            n300 = control-ref of="Modules Tree"() -> (w63:refnum<vi>)
            n301 = call "Set Tree custom symbols.vi"("TreeControl in"=w63) -> ("TreeControl out"=w62:refnum<vi>)  [unwired: 10 in]
          }
          event User Event {
            n302 = event-data() -> ("Projects"=w73:string[])  [unwired: 1 in]
            n303 = Array Size(array=w73) -> (size(s)=w72:i32)
            n304 = Equal?(x=1, y=w72) -> (x = y?=w70:bool)
            n305 = control-ref of="Projects"() -> (w74:refnum<vi>)
            n306 = case shown="False" w70 {
              tunnel: w74 -> [w80 w83]
              tunnel: w73 -> [w79 w82]
              frame True {
                n307 = Index Array(array=w79) -> (element=w78:string)  [unwired: 1 in]
                n308 = property class="CmbBox"(reference=w80, "Strings[]"=w79, "Val(Sgnl)"=w78) -> ()  [unwired: 1 in, 2 out]
              }
              frame False {
                n309 = property class="CmbBox"(reference=w83, "Strings[]"=w82, "Text.Text"="") -> ()  [unwired: 1 in, 2 out]
              }
            }
          }
          event User Event {
            n310 = event-data() -> ("Targets"=w85:string[])  [unwired: 1 in]
            n311 = Index Array(array=w85) -> (element=w84:string)  [unwired: 1 in]
            n312 = control-ref of="Targets"() -> (w87:refnum<vi>)
            n313 = property class="CmbBox"(reference=w87, "Strings[]"=w85, "Value"=w84) -> ()  [unwired: 1 in, 2 out]
          }
          event User Event {
            n314 = event-data() -> ("Progress"=→"Progress":u16)  [unwired: 1 in]
          }
          event Mouse Enter {
            n315 = event-data() -> ("CtlRef"=w94:refnum<vi>)  [unwired: 1 in]
            n316 = property class="Ctl"(reference=w94) -> ("Label.Text"=w99:string, "TipStrip"=w100:string)  [unwired: 1 in, 2 out]
            n317 = control-ref of="Panther Indicator"() -> (w98:refnum<vi>)
            n318 = control-ref of="Process Indicator"() -> (w97:refnum<vi>)
            n319 = control-ref of="Event Indicator"() -> (w96:refnum<vi>)
            n320 = Empty String/Path?(string/path=w100) -> (empty?=w101:bool)
            n321 = Build Array(w98, w97, w96) -> (w95:refnum<vi>[])
            n322 = call "Set Indicators Visibility Status.vi"("Indicator Refs"=w95, "Label"=w99) -> ()  [unwired: 10 in]
            n323 = case shown="False" w101 {
              tunnel: w100 -> [w105 _]
              frame False {
                n324 = call "Status Updated.vi"("Status"=w105) -> ()  [unwired: 10 in, 1 out]
              }
              frame True {
              }
            }
          }
          event User Event {
            n325 = event-data() -> ()  [unwired: 1 in, 1 out]
            n326 = control-ref of="This VI"() -> (w107:refnum<vi>)
            n327 = property class="VI"(reference=w107) -> ("Panel"=w108:refnum<vi>)  [unwired: 1 in, 2 out]
            n328 = property class="Pnl"(reference=w108) -> ("Controls[]"=w106:refnum<vi>[])  [unwired: 1 in, 2 out]
            n329 = register-events(reference=w111, w106) -> (reference out=w109:refnum<event-registration>)  [unwired: 3 in, 1 out]
          }
          event User Event {
            n330 = event-data() -> ("Scale Max"=w115:i32)  [unwired: 1 in]
            n331 = control-ref of="Progress"() -> (w114:refnum<vi>)
            n332 = property class="Slide (strict)"(reference=w114, "Scale.Maximum"=w115) -> (error out=w119:errorcluster)  [unwired: 1 in, 1 out]
          }
          event User Event {
            n333 = event-data() -> ("Module Type"=w126:T9)  [unwired: 1 in]
            n334 = Equal?(x=Module_type--enum."Module type: Cloneable", y=w126) -> (x = y?=w124:bool)
            n335 = Select(t=T12."Enabled" ("Disabled"), s=w124, f=T12."Disabled and Grayed Out") -> (s? t:f=w121:T12)
            n336 = control-ref of="Module ID"() -> (w123:refnum<vi>)
            n337 = property class="DigNum (strict)"(reference=w123, "DisabledEnum"=w121) -> ()  [unwired: 1 in, 2 out]
          }
          event User Event {
            n338 = event-data() -> ("Status"=→"Status":string)  [unwired: 1 in]
          }
        }
        n339 = call-dynamic "Delacor_lib_QMH_Error Handler - Helper Loop.vi"("error in"=w52, "Message Queue in"=w43) -> ("dup error in"=w51:errorcluster)  [unwired: 8 in, 1 out]
      }
    }
    frame Error {
      # "Synchronize Caller Events.vi will inform Start Module.vi that the module has launched and will let the code calling Start Module.vi register for broadcasts and would permit the caller receive the broadcast that an error occurred at launch time."
      n340 = call-dynamic "Delacor_lib_QMH_Release Message Queue.vi"("error in"=w777, "Message Queue"=w771) -> ("error out"=w776:errorcluster)  [unwired: 9 in]
      n341 = call "Synchronize Caller Events.vi"("Singleton Module Admin in"=w772) -> ("error out"=w778:errorcluster)  [unwired: 9 in, 1 out]
      n342 = call "Module Name--constant.vi"() -> ("Module Name"=w774:string)  [unwired: 11 in]
      n343 = Format Into String(format string="An error occurred during initialization. %s is no longer running.", w774) -> (resulting string=w769:string)  [unwired: 2 in, 1 out]
      n344 = Merge Errors(w776, w778) -> (w779:errorcluster)
      n345 = call "Stop Module.vi"("Origin"=w769) -> ()  [unwired: 10 in, 1 out]
      n346 = call "Error Reported.vi"("Additional Information"=w769, "Error"=w779) -> ()  [unwired: 9 in, 1 out]
    }
  }
  n347 = Merge Errors(w24, w26, w19) -> (w23:errorcluster)
  n348 = call "Close Module.vi"("error in (no error)"=w23, "Module Admin in"=w14) -> ("error out"=w25:errorcluster, "External Launch"=w8:bool, "Module Admin out"=w9:refnum<class "Delacor_lib_QMH_Module Admin.lvclass">)  [unwired: 7 in]
  n349 = Unregister For Events(event registration refnum=w6) -> ()  [unwired: 1 in, 1 out]
  n350 = Unregister For Events(event registration refnum=w13, error in=w25) -> (error out=w22:errorcluster)
  "error out" <- w22
  n351 = case "External Launch?" shown="True" w8 {
    tunnel: w22 -> [_ w780]
    frame False {
    }
    frame True {
      n352 = case shown="No Error" w780 {
        frame No Error {
          n353 = invoke class="VI" method="FP.Close"() -> ()  [unwired: 3 in, 3 out]
        }
        frame Error {
          n354 = invoke on="Invoke Node" class="VI" method="FP.Open"("Activate"=TRUE ("Activate?")) -> ()  [unwired: 4 in, 5 out]
        }
      }
    }
  }
  n355 = local write "Module Admin"(w9) -> ()
